vi "mul.vi"() -> ()   [LabVIEW 2013]
uses:
  <vilib>/Utility/config.llb/Read Key (String).vi
  <vilib>/Utility/config.llb/Write Key (String).vi
  <vilib>/Utility/config.llb/NI_LVConfig.lvlib
panel:
  in  "Boolean 2":bool caption="b2"
  out "Bindicator":bool caption="B1"
  in  "s1":string caption="s0"
  in  "Boolean":bool caption="B1"
  in  "Path":path caption="P1"
  out "String":string caption="s1"
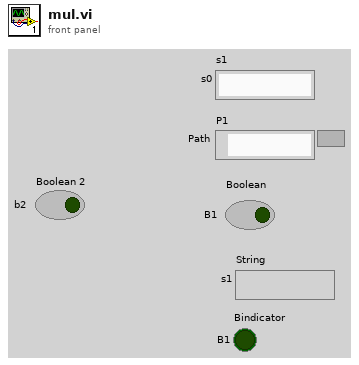
[diagram p1: front panel]
types:
  T1 = typedef "NI_LVConfig.lvlib/Config Data RefNum.ctl" = refnum<k1>
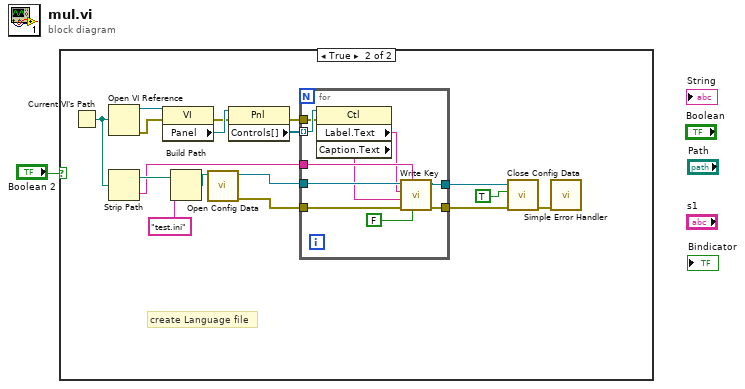
[diagram p0: block diagram]
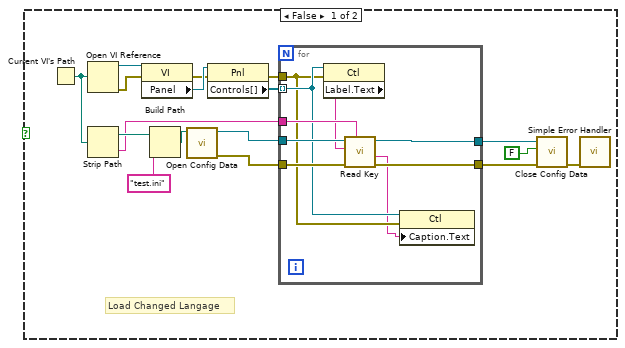
[diagram p2: hidden frame]
diagram:
  n1 = case shown="True" "Boolean 2" {
    frame False {
      # "Load Changed Langage"
      n2 = Current VI's Path() -> (path=w9:path)
      n3 = Open VI Reference(vi path=w9) -> (vi reference=w18:refnum<vi>, error out=w17:errorcluster)  [unwired: 5 in]
      n4 = Strip Path(path=w9) -> (stripped path=w13:path, name=w2:string)
      n5 = property class="VI"(reference=w18, error in=w17) -> (error out=w15:errorcluster, "Panel"=w16:refnum<vi>)  [unwired: 1 out]
      n6 = Build Path(base path=w13, name or relative path="test.ini") -> (appended path=w12:path)
      n7 = call <vilib>:"Open Config Data.vi"("configuration file path"=w12) -> ("error out"=w6:errorcluster, "refnum"=w7:T1)  [unwired: 8 in, 1 out]
      n8 = property class="Pnl"(reference=w16, error in=w15) -> (error out=w8:errorcluster, "Controls[]"=w14:refnum<vi>[])  [unwired: 1 out]
      n9 = for {
        tunnel: w14 -> [w21] mode=indexing
        tunnel: w8 -> [w20]
        tunnel: w7 -> [w27]
        tunnel: w6 -> [w26]
        tunnel: w2 -> [w25]
        tunnel: [w24] -> w5
        tunnel: [w23] -> w4
        n10 = property class="Ctl"(reference=w21, error in=w20) -> ("Label.Text"=w22:string)  [unwired: 2 out]
        n11 = call-poly <vilib>:"Read Key.vi"("section"=w25, "error in (no error)"=w26, "key"=w22, "refnum"=w27) -> ("error out"=w23:errorcluster, "value"=w19:string, "refnum out"=w24:T1)  [unwired: 4 in, 1 out]
        n12 = property class="Ctl"(reference=w21, error in=w20, "Caption.Text"=w19) -> ()  [unwired: 2 out]
      }
      n13 = call <vilib>:"Close Config Data.vi"("error in (no error)"=w4, "write file if changed (T)"=FALSE ("write configuration file? (T)"), "refnum"=w5) -> ("error out"=w11:errorcluster)  [unwired: 8 out]
      n14 = call <vilib>:"Simple Error Handler.vi"("error in (no error)"=w11) -> ()  [unwired: 1 in, 8 out]
    }
    frame True {
      # "create Language file"
      n15 = Current VI's Path() -> (path=w35:path)
      n16 = Open VI Reference(vi path=w35) -> (vi reference=w44:refnum<vi>, error out=w43:errorcluster)  [unwired: 5 in]
      n17 = Strip Path(path=w35) -> (stripped path=w39:path, name=w28:string)
      n18 = property class="VI"(reference=w44, error in=w43) -> (error out=w41:errorcluster, "Panel"=w42:refnum<vi>)  [unwired: 1 out]
      n19 = Build Path(base path=w39, name or relative path="test.ini") -> (appended path=w38:path)
      n20 = call <vilib>:"Open Config Data.vi"("configuration file path"=w38) -> ("error out"=w32:errorcluster, "refnum"=w33:T1)  [unwired: 8 in, 1 out]
      n21 = property class="Pnl"(reference=w42, error in=w41) -> (error out=w34:errorcluster, "Controls[]"=w40:refnum<vi>[])  [unwired: 1 out]
      n22 = for {
        tunnel: w40 -> [w54] mode=indexing
        tunnel: w34 -> [w53]
        tunnel: w33 -> [w52]
        tunnel: w32 -> [w51]
        tunnel: w28 -> [w50]
        tunnel: [w49] -> w31
        tunnel: [w48] -> w30
        n23 = property class="Ctl"(reference=w54, error in=w53) -> ("Label.Text"=w46:string, "Caption.Text"=w45:string)  [unwired: 2 out]
        n24 = call-poly <vilib>:"Write Key.vi"("write raw string? (F)"=FALSE, "section"=w50, "error in (no error)"=w51, "value"=w45, "key"=w46, "refnum"=w52) -> ("error out"=w48:errorcluster, "refnum out"=w49:T1)  [unwired: 3 in, 1 out]
      }
      n25 = call <vilib>:"Close Config Data.vi"("error in (no error)"=w30, "write file if changed (T)"=TRUE ("write configuration file? (T)"), "refnum"=w31) -> ("error out"=w37:errorcluster)  [unwired: 8 out]
      n26 = call <vilib>:"Simple Error Handler.vi"("error in (no error)"=w37) -> ()  [unwired: 1 in, 8 out]
    }
  }
